vi "INI_Driver.vi"(0 "Data_In":string, 1 "Config_File_Path":path, 11 "Error_Out":errorcluster, 13 "INI_Operation_Select":T1=enum."Write") -> (4 "Data_Out":string, 15 "Error_Out":errorcluster)   [LabVIEW 2023]
doc: "Used to read and write the ini file"
uses:
  Controls/INI_Operation_Select.ctl
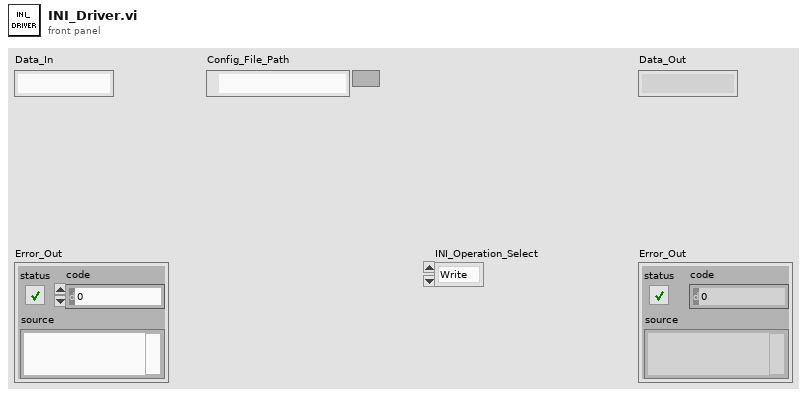
[diagram p1: front panel]
types:
  T1 = typedef "INI_Operation_Select.ctl" = enum16{"Initialize", "Read", "Read_Key", "Write"}
  T2 = enum16{"open", "replace", "create", "open or create", "replace or create", "replace or create with confirmation"}
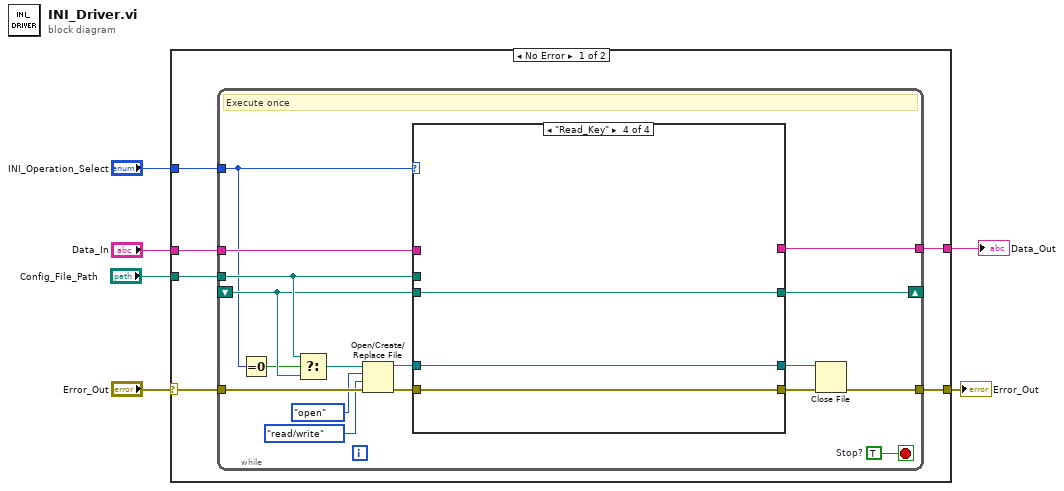
[diagram p0: block diagram]
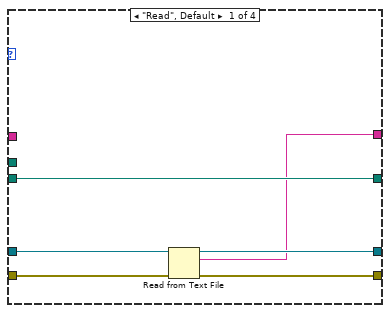
[diagram p2: hidden frame]
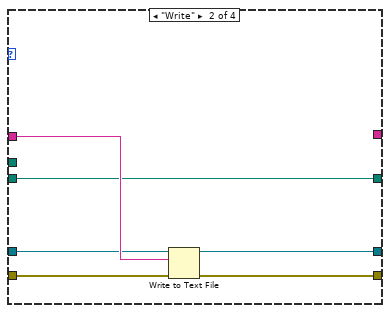
[diagram p3: hidden frame]
diagram:
  n1 = case shown="No Error" "Error_Out" {
    selector: "Error_Out" -> [w10 w48]
    tunnel: "INI_Operation_Select" -> [w12 _]
    tunnel: [w11 w48] -> w4
    tunnel: [w9 _] -> w3
    tunnel: "Data_In" -> [w8 _]
    tunnel: "Config_File_Path" -> [w7 _]
    frame No Error {
      n2 = while {
        tunnel: w12 -> [w16]
        tunnel: [w21] -> w11
        tunnel: w10 -> [w25]
        tunnel: [w28] -> w9
        tunnel: w8 -> [w27]
        shift-right: [w20] -> _
        shift-left: _ -> [w17]
        tunnel: w7 -> [w18]
        stop <- w29 stop-if-true
        w29 = TRUE  # Stop?
        # "Execute once"
        n3 = Equal To 0?(x=w16) -> (x = 0?=w15:bool)
        n4 = Select(t=w18, s=w15, f=w17) -> (s? t:f=w19:path)
        n5 = Open/Create/Replace File(file path (use dialog)=w19, error in=w25, operation (0:open)=T2."open", access (0:read/write)=enum16{"read/write", "read-only", "write-only"}."read/write") -> (refnum out=w26:refnum<file>, error out=w24:errorcluster)  [unwired: 2 in, 1 out]
        n6 = case shown="\"Read_Key\"" w16 {
          tunnel: [w32 w39 w44 w46] -> w22
          tunnel: w24 -> [w34 w40 w44 w46]
          tunnel: [w30 _ _ _] -> w28
          tunnel: w27 -> [_ w41 _ _]
          tunnel: w18 -> [_ _ w43 _]
          tunnel: w26 -> [w35 w36 w42 w45]
          tunnel: [w33 w38 w42 w45] -> w23
          tunnel: [w31 w37 w43 w47] -> w20
          tunnel: w17 -> [w31 w37 _ w47]
          frame "Read", Default {
            n7 = Read from Text File(file (use dialog)=w35, error in=w34) -> (refnum out=w33:refnum<file>, text=w30:string, error out=w32:errorcluster)  [unwired: 2 in, 1 out]
          }
          frame "Write" {
            n8 = Write to Text File(file (use dialog)=w36, text=w41, error in=w40) -> (refnum out=w38:refnum<file>, error out=w39:errorcluster)  [unwired: 1 in, 1 out]
          }
          frame "Initialize" {
          }
          frame "Read_Key" {
          }
        }
        n9 = Close File(refnum=w23, error in=w22) -> (error out=w21:errorcluster)  [unwired: 1 out]
      }
    }
    frame Error {
    }
  }
  "Error_Out" <- w4
  "Data_Out" <- w3
